vi "ex2_4b.vi"() -> ()   [LabVIEW 2017]
panel:
  out "DIODE VI CHARACTERISTICS":cluster{"Y":dbl[], "Y":dbl[]}[](graph)
  out "VI curve of LM 4007 diode":cluster{dbl[], dbl[]}(graph)
  out "Measured voltage":dbl
  out "Measured current":dbl
  in  "Applied resistance (Ohm)":dbl
  in  "stop":bool
  in  "Step size":dbl=0.01
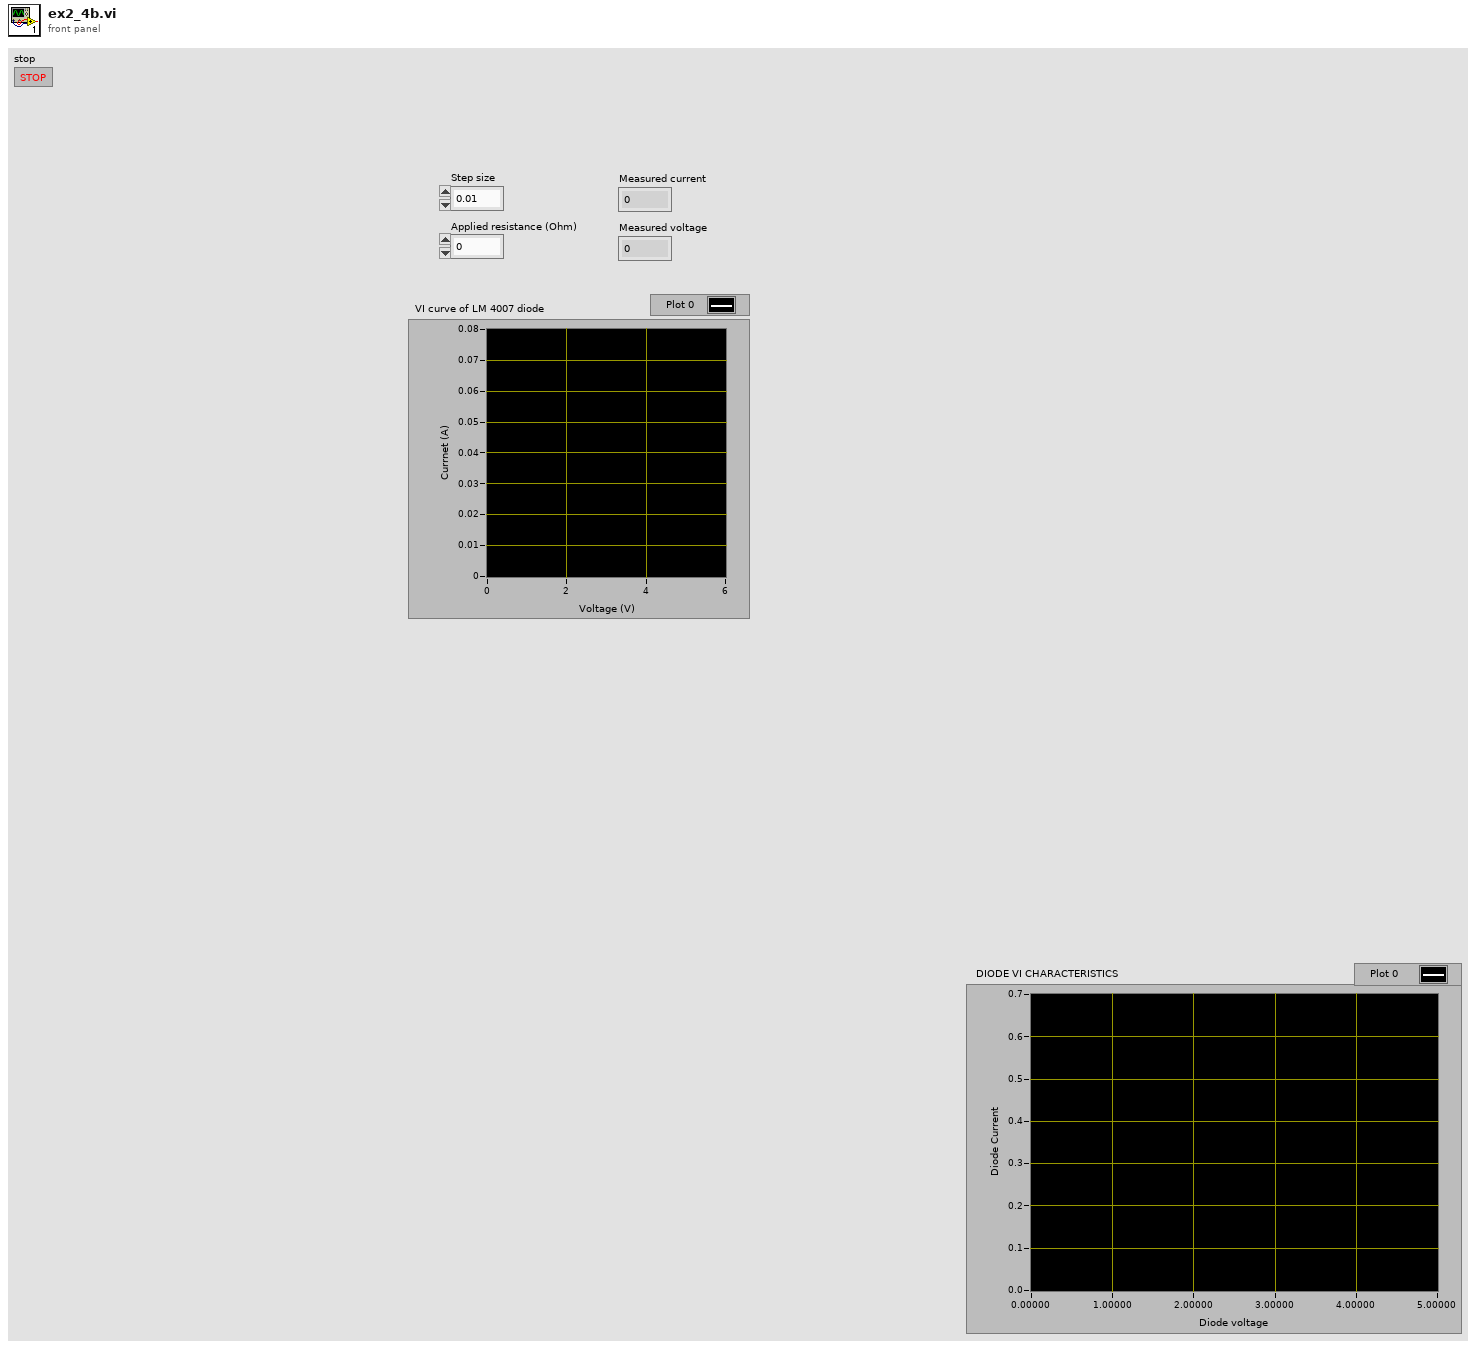
[diagram p1: front panel]
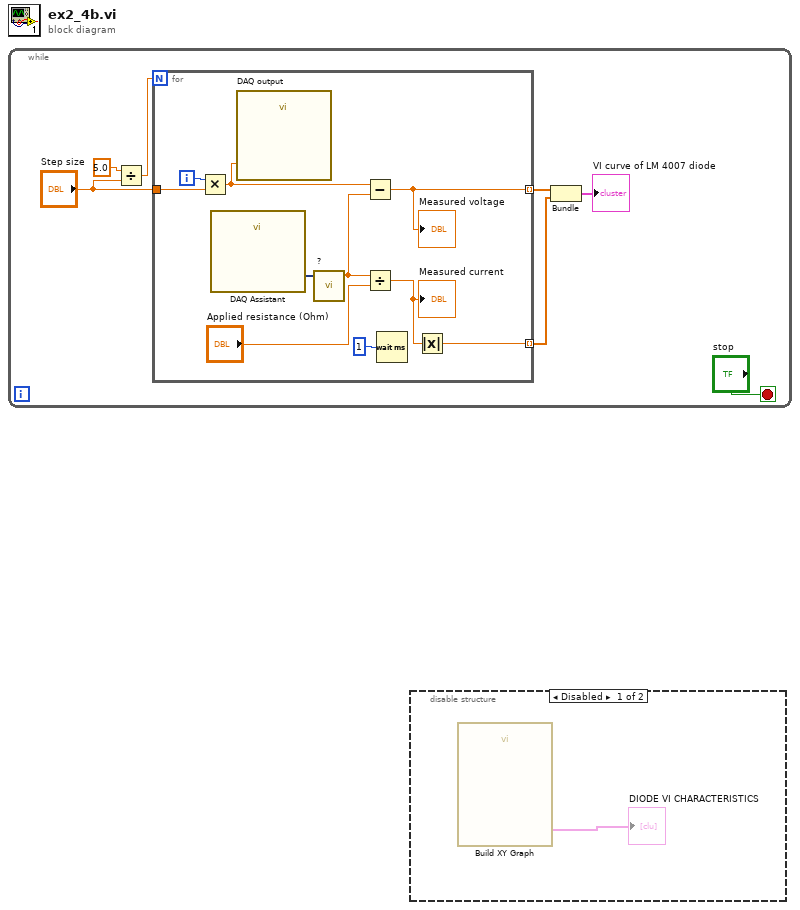
[diagram p0: block diagram]
diagram:
  n1 = while {
    stop <- "stop" stop-if-true
    n2 = Divide(x=5.0, y="Step size") -> (x/y=w6:dbl)
    n3 = for {
      N: w6 -> [_]
      tunnel: "Step size" -> [w16]
      tunnel: [w8] -> w1 mode=indexing
      tunnel: [w12] -> w2 mode=indexing
      i -> [w17]
      n4 = Multiply(x=w17, y=w16) -> (x*y=w13:dbl)
      n5 = call "DAQ Assistant"() -> ("data"=w15:dynamicdata)  [unwired: 17 in, 2 out]
      n6 = call "DAQ output"("data"=w13) -> ()  [unwired: 17 in, 2 out]
      n7 = call "?"("Dynamic Data Type"=w15) -> ("Scalar"=w10:dbl)  [unwired: 3 in]
      n8 = Subtract(x=w13, y=w10) -> (x-y=w12:dbl)
      "Measured voltage" <- w12
      n9 = Divide(x=w10, y="Applied resistance (Ohm)") -> (x/y=w9:dbl)
      "Measured current" <- w9
      n10 = Wait (ms)(milliseconds to wait=u32 1) -> ()  [unwired: 1 out]
      n11 = Absolute Value(x=w9) -> (abs(x)=w8:dbl)
    }
    n12 = Bundle(w2, w1) -> (→"VI curve of LM 4007 diode":cluster{dbl[], dbl[]})  [unwired: 1 in]
  }
  n13 = disable-structure shown="Disabled" {
    frame Disabled {
      n14 = call "Build XY Graph"() -> ("XY Graph"=→"DIODE VI CHARACTERISTICS":cluster{"X":dbl[], "Y":dbl[]}[])  [unwired: 10 in, 1 out]
    }
    frame Enabled {
    }
  }
